vi "Write measurement type.vi"(8 "error in (no error)":errorcluster, 10 "measurement type (voltage)":i32(ring)=1 items=["Voltage"=1, "Current"=0], 11 "Measure [MSR] Msg in":refnum<class "Measure [MSR] Msg.lvclass">) -> (0 "error out":errorcluster, 3 "Measure [MSR] Msg out":refnum<class "Measure [MSR] Msg.lvclass">)   [LabVIEW 2013, in "CS++DCPwr.lvlib" / "Measure [MSR] Msg.lvclass"]
uses:
  Measure [MSR] Msg.lvclass
  Measure [MSR] Msg.lvclass/Measure [MSR] Msg.ctl
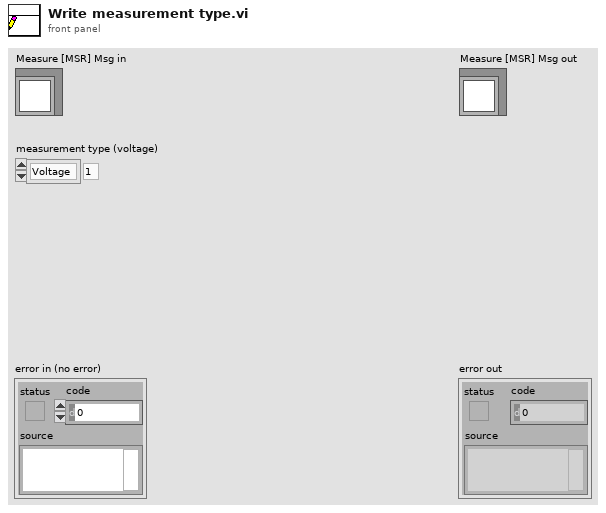
[diagram p1: front panel]
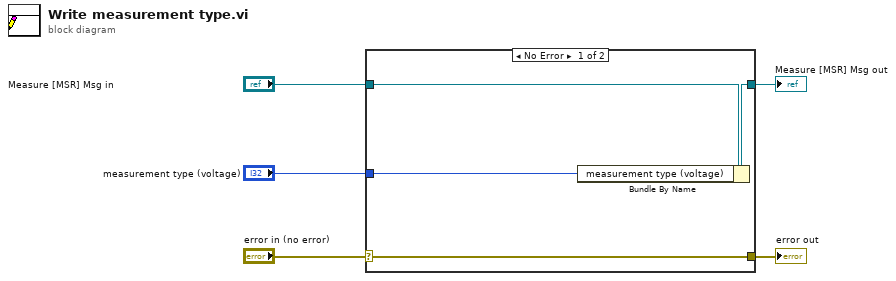
[diagram p0: block diagram]
diagram:
  n1 = case shown="No Error" "error in (no error)" {
    selector: "error in (no error)" -> [w9 w10]
    tunnel: [w9 w10] -> w4
    tunnel: [w7 w11] -> w2
    tunnel: "Measure [MSR] Msg in" -> [w8 w11]
    tunnel: "measurement type (voltage)" -> [w6 _]
    frame No Error {
      n2 = Bundle By Name(cluster=w8, "measurement type (voltage)"=w6) -> (w7:refnum<class "Measure [MSR] Msg.lvclass">)
    }
    frame Error {
    }
  }
  "error out" <- w4
  "Measure [MSR] Msg out" <- w2
